vi "Read Trace (Occupied Bandwidth).vi"(8 "error in (no error)":errorcluster, 10 "Timeout (10000 ms)":i32=10000 format="%.0g", 11 "VISA resource name":refnum<visa-resource-name>) -> (0 "error out":errorcluster, 2 "Trace Waveform":T1(graph), 3 "VISA resource name out":refnum<visa-resource-name>)   [LabVIEW 2014, in "Agilent MXA Series.lvlib"]
doc: "Reads the trace from the spectrum analyzer(Occupied Bandwidth)."
uses:
  Agilent MXA Series.lvlib
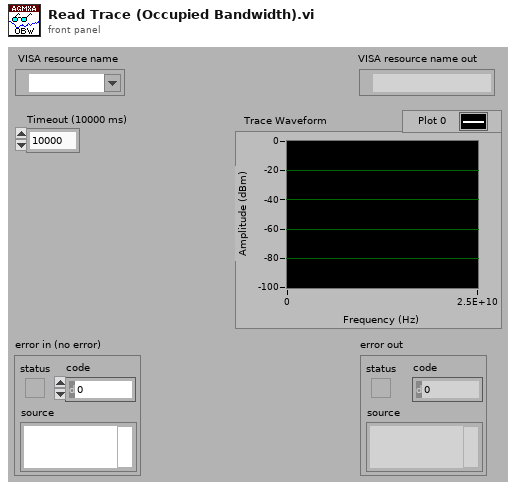
[diagram p1: front panel]
types:
  T1 = cluster{"Initial X":dbl, "X Increment":dbl, "Trace Array":dbl[]}
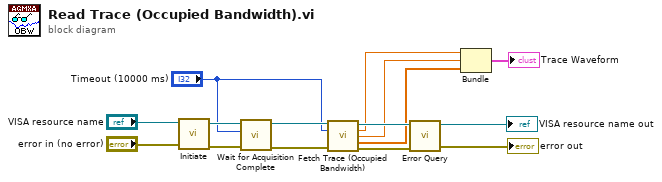
[diagram p0: block diagram]
diagram:
  n1 = call "Initiate.vi"("error in (no error)"="error in (no error)", "VISA resource name"="VISA resource name") -> ("error out"=w12:errorcluster, "VISA resource name out"=w13:refnum<visa-resource-name>)  [unwired: 8 in]
  n2 = call "Wait for Acquisition Complete.vi"("error in (no error)"=w12, "Maximum Time (10000)"="Timeout (10000 ms)", "VISA resource name"=w13) -> ("error out"=w10:errorcluster, "VISA resource name out"=w11:refnum<visa-resource-name>)  [unwired: 7 in]
  n3 = call "Fetch Trace (Occupied Bandwidth).vi"("VISA resource name"=w11, "Timeout (10000 ms)"="Timeout (10000 ms)", "error in (no error)"=w10) -> ("VISA resource name out"=w9:refnum<visa-resource-name>, "Initial X"=w4:dbl, "X Increment"=w3:dbl, "Trace Array"=w2:dbl[], "error out"=w8:errorcluster)  [unwired: 8 in]
  n4 = call "Error Query.vi"("error in (no error)"=w8, "VISA resource name"=w9) -> ("error out"=→"error out":errorcluster, "VISA resource name out"=→"VISA resource name out":refnum<visa-resource-name>)  [unwired: 6 in, 2 out]
  n5 = Bundle("Initial X"=w4, "X Increment"=w3, "Trace Array"=w2) -> (→"Trace Waveform":T1)  [unwired: 1 in]
